vi "Create.vi"(8 "error in (no error)":errorcluster, 9 "Movie Settings":T1={"Camera Settings"={"Exposure Time (ms)"=100.0, "Binning"=enum."2x2", "Scan Mode"=0, "Frames to Acquire"=1000.0, "Pixel Correction"=FALSE, "Frames to Skip"=0, "File Path"=path "", "Duty cycle"=0.0, "ALEX"=FALSE, "Shutter Enable"=[], "fluidics trigger, ms (0=disabled)"=0.0, "Bit Depth"=0, "Image Width (px)"=0, "Image Height (px)"=0, "Horizontal Offset (px)"=0, "Vertical Offset (px)"=0}, "Auto-Advance"=TRUE, "Auto Focus"=TRUE, "Injection Countdown"=TRUE, "Laser Power (mW)"=0, "Termination Criteria"={"Particle Count Threshold"=0, "Min Frames"=0}} {"Camera Settings"."Exposure Time (ms)" min=1.0 max=10000.0 step=1.0}, 10 "Movie Series":T3={"Fields"=1, "Lanes"=1, "Acquisition type"=enum."Movie series", "Sweeps"=[]}) -> (0 "error out":errorcluster, 3 "Protocol out":refnum<class "Protocol.lvclass">)   [LabVIEW 2023, in "Automation.lvlib" / "Protocol.lvclass"]
uses:
  Protocol.lvclass
  Resources/Type Defs/Movie Series.ctl
  Resources/Type Defs/Movie auto-numbering.ctl
  Resources/Type Defs/Param Sweep.ctl
  Resources/Type Defs/Sweep Parameter.ctl
  Resources/Type Defs/Movie Settings.ctl
  Resources/Type Defs/Camera Settings.ctl
  Protocol.lvclass/Protocol.ctl
panel:
  in  "Protocol in":refnum<class "Protocol.lvclass">
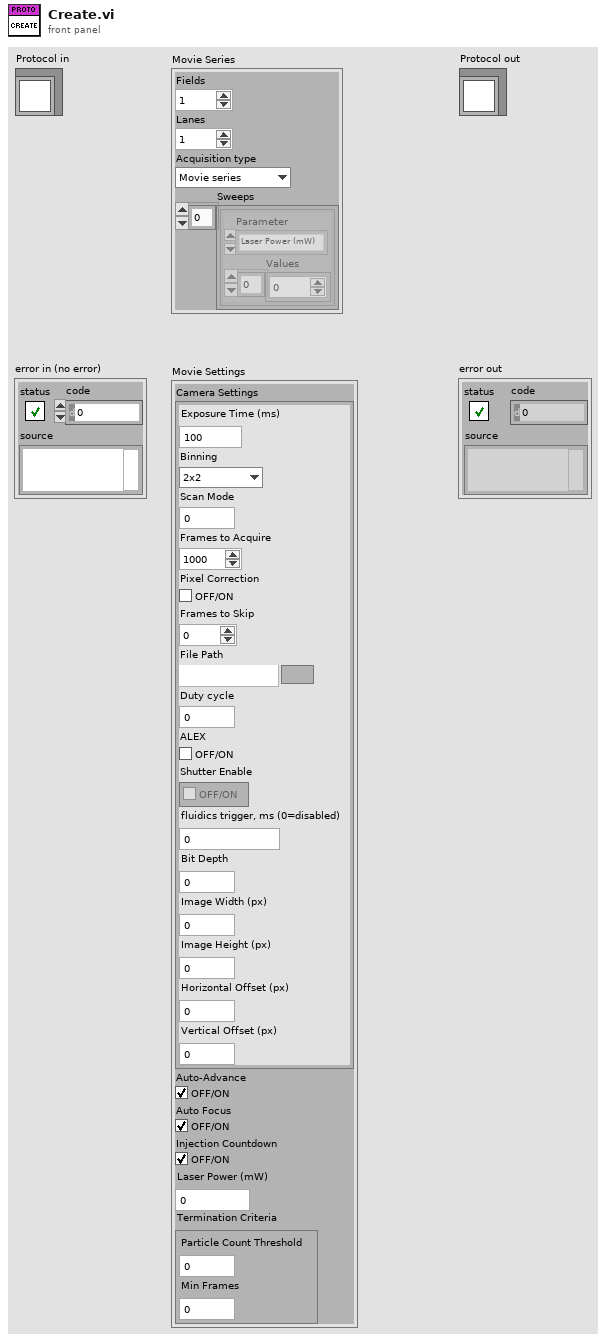
[diagram p1: front panel]
types:
  T1 = typedef "Movie Settings.ctl" = cluster{"Camera Settings":T2, "Auto-Advance":bool, "Auto Focus":bool, "Injection Countdown":bool, "Laser Power (mW)":u32, "Termination Criteria":cluster{"Particle Count Threshold":i32, "Min Frames":i32}}
  T2 = typedef "Camera Settings.ctl" = cluster{"Exposure Time (ms)":dbl, "Binning":enum16{"1x1", "2x2", "4x4"}, "Scan Mode":i32, "Frames to Acquire":dbl, "Pixel Correction":bool, "Frames to Skip":u32, "File Path":path, "Duty cycle":dbl, "ALEX":bool, "Shutter Enable":bool[], "fluidics trigger, ms (0=disabled)":dbl, "Bit Depth":u16, "Image Width (px)":u16, "Image Height (px)":u16, "Horizontal Offset (px)":u16, "Vertical Offset (px)":u16}
  T3 = typedef "Movie Series.ctl" = cluster{"Fields":i32, "Lanes":i32, "Acquisition type":T4, "Sweeps":T5[]}
  T4 = typedef "Movie auto-numbering.ctl" = enum16{"Single movie", "Movie series", "Multi-lane series", "Sweep Parameter"}
  T5 = typedef "Param Sweep.ctl" = cluster{"Parameter":T6, "Values":u32[]}
  T6 = typedef "Sweep Parameter.ctl" = enum16{"Laser Power (mW)", "Exposure Time (ms)", "Number of Frames", "Laser Line (1,2,3,4)"}
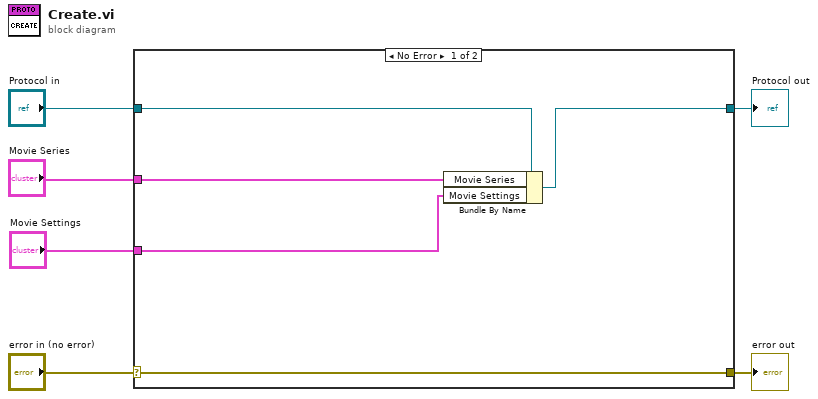
[diagram p0: block diagram]
diagram:
  n1 = case shown="No Error" "error in (no error)" {
    selector: "error in (no error)" -> [w11 w13]
    tunnel: [w11 w13] -> w5
    tunnel: [w9 w12] -> w3
    tunnel: "Protocol in" -> [w10 w12]
    tunnel: "Movie Series" -> [w8 _]
    tunnel: "Movie Settings" -> [w7 _]
    frame No Error {
      n2 = Bundle By Name(cluster=w10, "Movie Series"=w8, "Movie Settings"=w7) -> (w9:refnum<class "Protocol.lvclass">)
    }
    frame Error {
    }
  }
  "error out" <- w5
  "Protocol out" <- w3
